vi "ReadContinuous.vi"(8 "error in (no error)":errorcluster, 10 "Qbus in":refnum<class "Qbus.lvclass">, 11 "config":T1) -> (0 "error out":errorcluster, 2 "next action":string, 3 "cofig out":T1)   [LabVIEW 2017, in "EmsaAcquisition.lvlib"]
uses:
  <vilib>/addons/InsightCM/Devices/Shared/Emsa/EmsaAcquisition/EmsaAcquisition.lvlib
  <vilib>/addons/Qbus/Qbus.lvclass
  <vilib>/addons/InsightCM/Devices/Shared/Emsa/EmsaAcquisition/controls/config.ctl
  <vilib>/addons/InsightCM/Devices/Shared/Emsa/Emsa9770API/9770 API.lvclass
  <vilib>/addons/InsightCM/Devices/Shared/Emsa/EmsaAcquisition/controls/group.ctl
  <vilib>/addons/InsightCM/Devices/Shared/Emsa/EmsaAcquisition/controls/acqConfig.ctl
  <vilib>/addons/InsightCM/Devices/Shared/Emsa/EmsaAcquisition/controls/OnDemandWaveformData.ctl
  <vilib>/measure/NI_MAPro.lvlib
  <vilib>/measure/macond.llb/IIR Filter for 1 Chan (CDB).vi
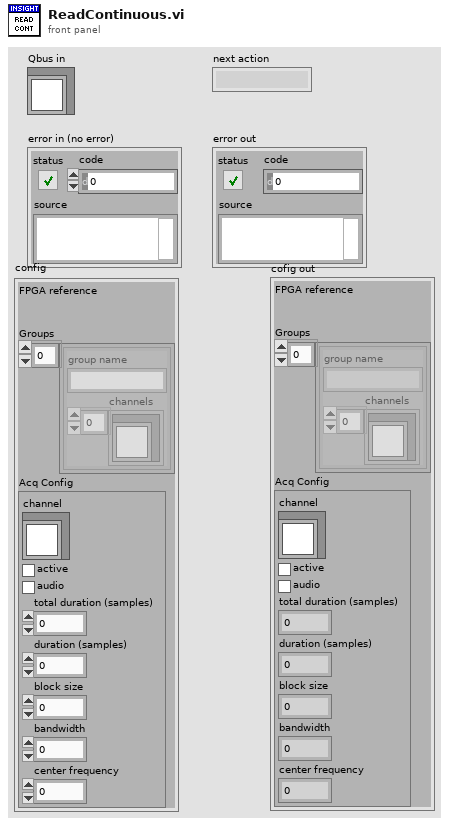
[diagram p1: front panel]
types:
  T1 = typedef "EmsaAcquisition.lvlib/config.ctl" = cluster{"FPGA reference":refnum<k20>, "Groups":T2[], "Acq Config":T3}
  T2 = typedef "EmsaAcquisition.lvlib/group.ctl" = cluster{"group name":string, "channels":refnum<class "9770 API.lvclass">[]}
  T3 = typedef "EmsaAcquisition.lvlib/acqConfig.ctl" = cluster{"channel":refnum<class "9770 API.lvclass">, "active":bool, "audio":bool, "total duration (samples)":i32, "duration (samples)":i32, "block size":i32, "bandwidth":dbl, "center frequency":dbl}
  T4 = typedef "EmsaAcquisition.lvlib/OnDemandWaveformData.ctl" = cluster{"Channel":string, "First Block":bool, "Last Block":bool, "Center Frequency":dbl, "Waveform":waveform(dbl)}
  T5 = cluster{"Topology":enum16{"Off", "Butterworth", "Chebyshev", "Inverse Chebyshev", "Elliptic", "Bessel"}, "Type":enum16{"Lowpass", "Highpass", "Bandpass", "Bandstop"}, "Order":i32, "Lower Fc":dbl, "Upper Fc":dbl, "PB Ripple":dbl, "SB Attenuation":dbl}
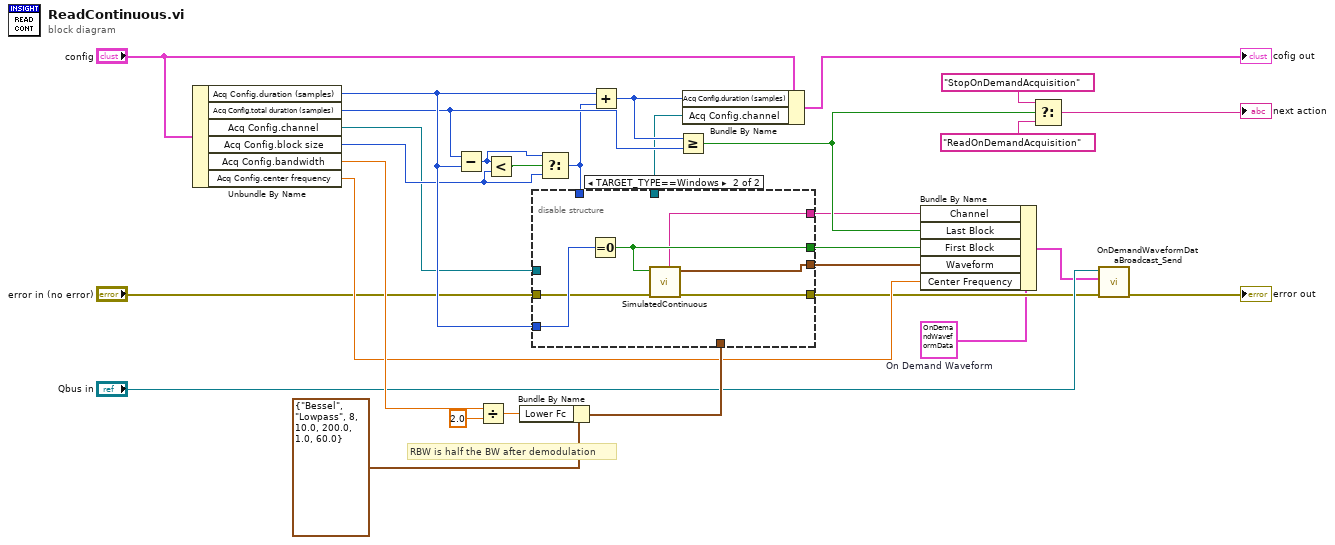
[diagram p0: block diagram]
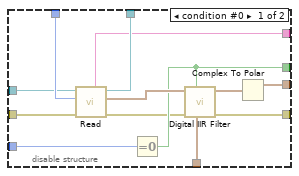
[diagram p2: hidden frame]
diagram:
  w1 = T4 {"Channel"="", "First Block"=FALSE, "Last Block"=FALSE, "Center Frequency"=0.0, "Waveform"={"t0"=timestamp(0 s since 1904-01-01), "dt"=1.0, "Y"=[]}}  # On Demand Waveform
  # "RBW is half the BW after demodulation"
  n1 = Unbundle By Name("config") -> ("Acq Config.duration (samples)"=w22:i32, "Acq Config.total duration (samples)"=w15:i32, "Acq Config.channel"=w8:refnum<class "9770 API.lvclass">, "Acq Config.block size"=w11:i32, "Acq Config.bandwidth"=w28:dbl, "Acq Config.center frequency"=w23:dbl)
  n2 = Subtract(x=w15, y=w22) -> (x-y=w12:i32)
  n3 = Divide(x=w28, y=2.0) -> (x/y=w27:dbl)
  n4 = Less?(x=w12, y=w11) -> (x < y?=w10:bool)
  n5 = Bundle By Name(cluster=T5 {"Topology"=enum."Bessel", "Type"=enum."Lowpass", "Order"=8, "Lower Fc"=10.0, "Upper Fc"=200.0, "PB Ripple"=1.0, "SB Attenuation"=60.0} ("IIR filter specifications"), "Lower Fc"=w27) -> (w25:T5)
  n6 = Select(t=w12, s=w10, f=w11) -> (s? t:f=w13:i32)
  n7 = disable-structure shown="TARGET_TYPE==Windows" {
    disable-tunnel: [w42 w45] -> w30
    disable-tunnel: [w40 w46] -> w26
    disable-tunnel: w25 -> [w39 _]
    disable-tunnel: w22 -> [w38 w49]
    disable-tunnel: w13 -> [w37 _]
    disable-tunnel: [w36 _] -> w9
    disable-tunnel: w8 -> [w35 _]
    disable-tunnel: "error in (no error)" -> [w34 w48]
    disable-tunnel: [w32 w47] -> w4
    disable-tunnel: [w31 w44] -> w3
    frame condition #0 {
      n8 = call <vilib>:"Read.vi"("error in (no error)"=w34, "number of samples"=w37, "9770 API in"=w35) -> ("error out"=w33:errorcluster, "Waveform"=w43:waveform(cdb), "9770 API out"=w36:refnum<class "9770 API.lvclass">, "ChannelName"=w31:string)  [unwired: 3 in, 2 out]
      n9 = Equal To 0?(x=w38) -> (x = 0?=w40:bool)
      n10 = call-poly <vilib>:"Digital IIR Filter.vi"("IIR filter specifications"=w39, "reset filter"=w40, "error in (no error)"=w33, "signal in"=w43) -> ("error out"=w32:errorcluster, "signal out"=w41:waveform(cdb))  [unwired: 5 in, 1 out]
      n11 = Complex To Polar(r * e^(i*theta)=w41) -> (r=w42:waveform(dbl))  [unwired: 1 out]
    }
    frame condition #1 (active) {
      n12 = Equal To 0?(x=w49) -> (x = 0?=w46:bool)
      n13 = call <vilib>:"SimulatedContinuous.vi"("error in (no error)"=w48, "first block"=w46) -> ("error out"=w47:errorcluster, "signal out"=w45:waveform(dbl), "Channel"=w44:string)  [unwired: 7 in]
    }
  }
  n14 = Add(x=w22, y=w13) -> (x+y=w14:i32)
  n15 = Greater Or Equal?(x=w14, y=w15) -> (x >= y?=w21:bool)
  n16 = Bundle By Name(cluster="config", "Acq Config.duration (samples)"=w14, "Acq Config.channel"=w9) -> (→"cofig out":T1)
  n17 = Bundle By Name(cluster=w1, "Channel"=w3, "Last Block"=w21, "First Block"=w26, "Waveform"=w30, "Center Frequency"=w23) -> (w2:T4)
  n18 = Select(t="StopOnDemandAcquisition", s=w21, f="ReadOnDemandAcquisition") -> (s? t:f=→"next action":string)
  n19 = call <vilib>:"OnDemandWaveformDataBroadcast_Send.vi"("error in (no error)"=w4, "On Demand Waveform"=w2, "Qbus"="Qbus in") -> ("error out"=→"error out":errorcluster)  [unwired: 7 in, 1 out]
